vi "Build Description String.vi"(8 "error in (no error)":errorcluster, 11 "String Assertion in":refnum<class "String Assertion.lvclass">) -> (0 "error out":errorcluster, 2 "Description":string, 3 "String Assertion out":refnum<class "String Assertion.lvclass">)   [LabVIEW 2020, in "MacroAssert.lvlib" / "String Assertion.lvclass"]
doc: "Builds a string to describe what <B>Step</B> does."
uses:
  String Assertion.lvclass
  Assertion Step/Assertion Step.lvclass
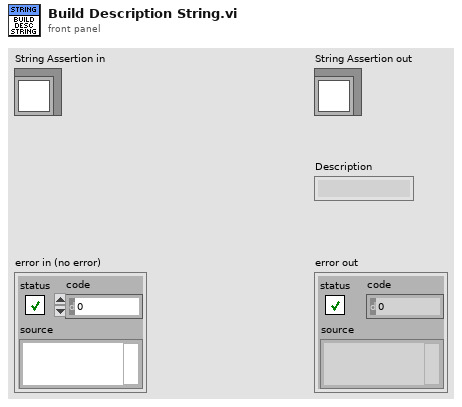
[diagram p1: front panel]
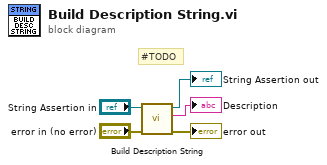
[diagram p0: block diagram]
diagram:
  # "#TODO"
  n1 = call-parent "Build Description String.vi"("error in (no error)"="error in (no error)", "Step in"="String Assertion in") -> ("error out"=→"error out":errorcluster, "Description"=→"Description":string, "Step out"=→"String Assertion out":refnum<class "String Assertion.lvclass">)  [unwired: 7 in]
